vi "Volts_to_temperature_(SubVI).vi"(4 "input variable":i32, 7 "error in":errorcluster, 16 "koeff. cluster":T1) -> (20 "T solvation":dbl, 21 "meas_voltage":dbl, 27 "error out":errorcluster)   [LabVIEW 2015]
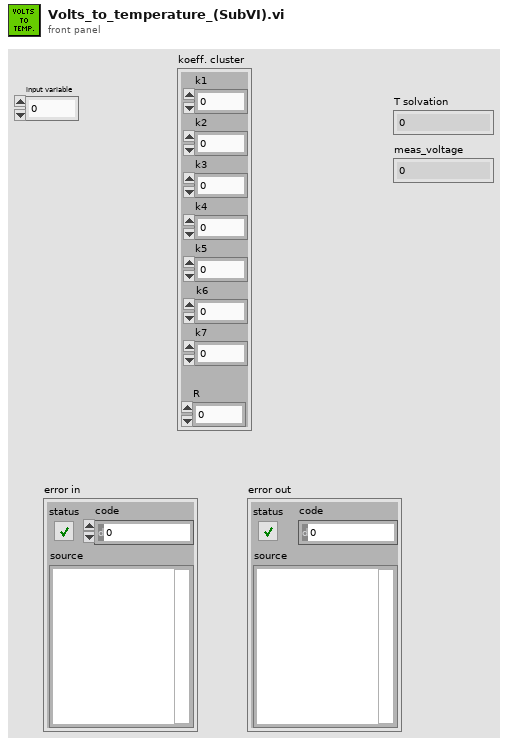
[diagram p1: front panel]
types:
  T1 = cluster{"k1":ext, "k2":ext, "k3":ext, "k4":ext, "k5":ext, "k6":ext, "k7":ext, "R":ext}
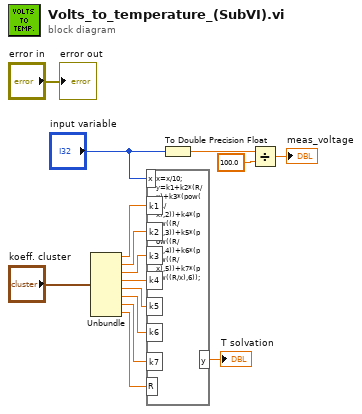
[diagram p0: block diagram]
diagram:
  n1 = Unbundle("koeff. cluster") -> ("k1"=w11:ext, "k2"=w9:ext, "k3"=w8:ext, "k4"=w7:ext, "k5"=w6:ext, "k6"=w5:ext, "k7"=w4:ext, "R"=w10:ext)
  n2 = formula code="x=x/10;\ny=k1+k2*(R/x)+k3*(pow((R/x),2))+k4*(pow((R/x),3))+k5*(pow((R/x),4))+k6*(pow((R/x),5))+k7*(pow((R/x),6));"("x"="input variable", "k1"=w11, "k2"=w9, "k3"=w8, "k4"=w7, "k5"=w6, "k6"=w5, "k7"=w4, "R"=w10) -> ("y"=→"T solvation":dbl)
  n3 = To Double Precision Float(number="input variable") -> (double precision float=w1:dbl)
  n4 = Divide(x=w1, y=100.0) -> (x/y=→"meas_voltage":dbl)
  "error out" <- "error in"
